vi "Compare to masks.vi"(7 "Number of Particles1":i32=10, 8 "error in (no error)":errorcluster, 9 "Number of Particles":i32=1, 10 "Mask array":T1[](array[typedef]), 11 "Image Src":T1=refnum) -> (0 "Final error out":errorcluster={"status"=TRUE, "code"=-1074395995, "source"=""}, 3 "Marked Regions":bool[](array[boolean]))   [LabVIEW 2009]
doc: "From the marked regions, this VI outputs a one dimensional array of integers. Each element is a sector with a sick distance value in it. The 0th element represents the sector at 180 degrees, whlie the 29th element represents the sector at 0 degrees"
uses:
  <vilib>/vision/Image Controls.llb/IMAQ Image.ctl
  <vilib>/vision/NI_Vision_Development_Module.lvlib
panel:
  out "x < 0?":bool
  out "Erosion iteration":i32=3
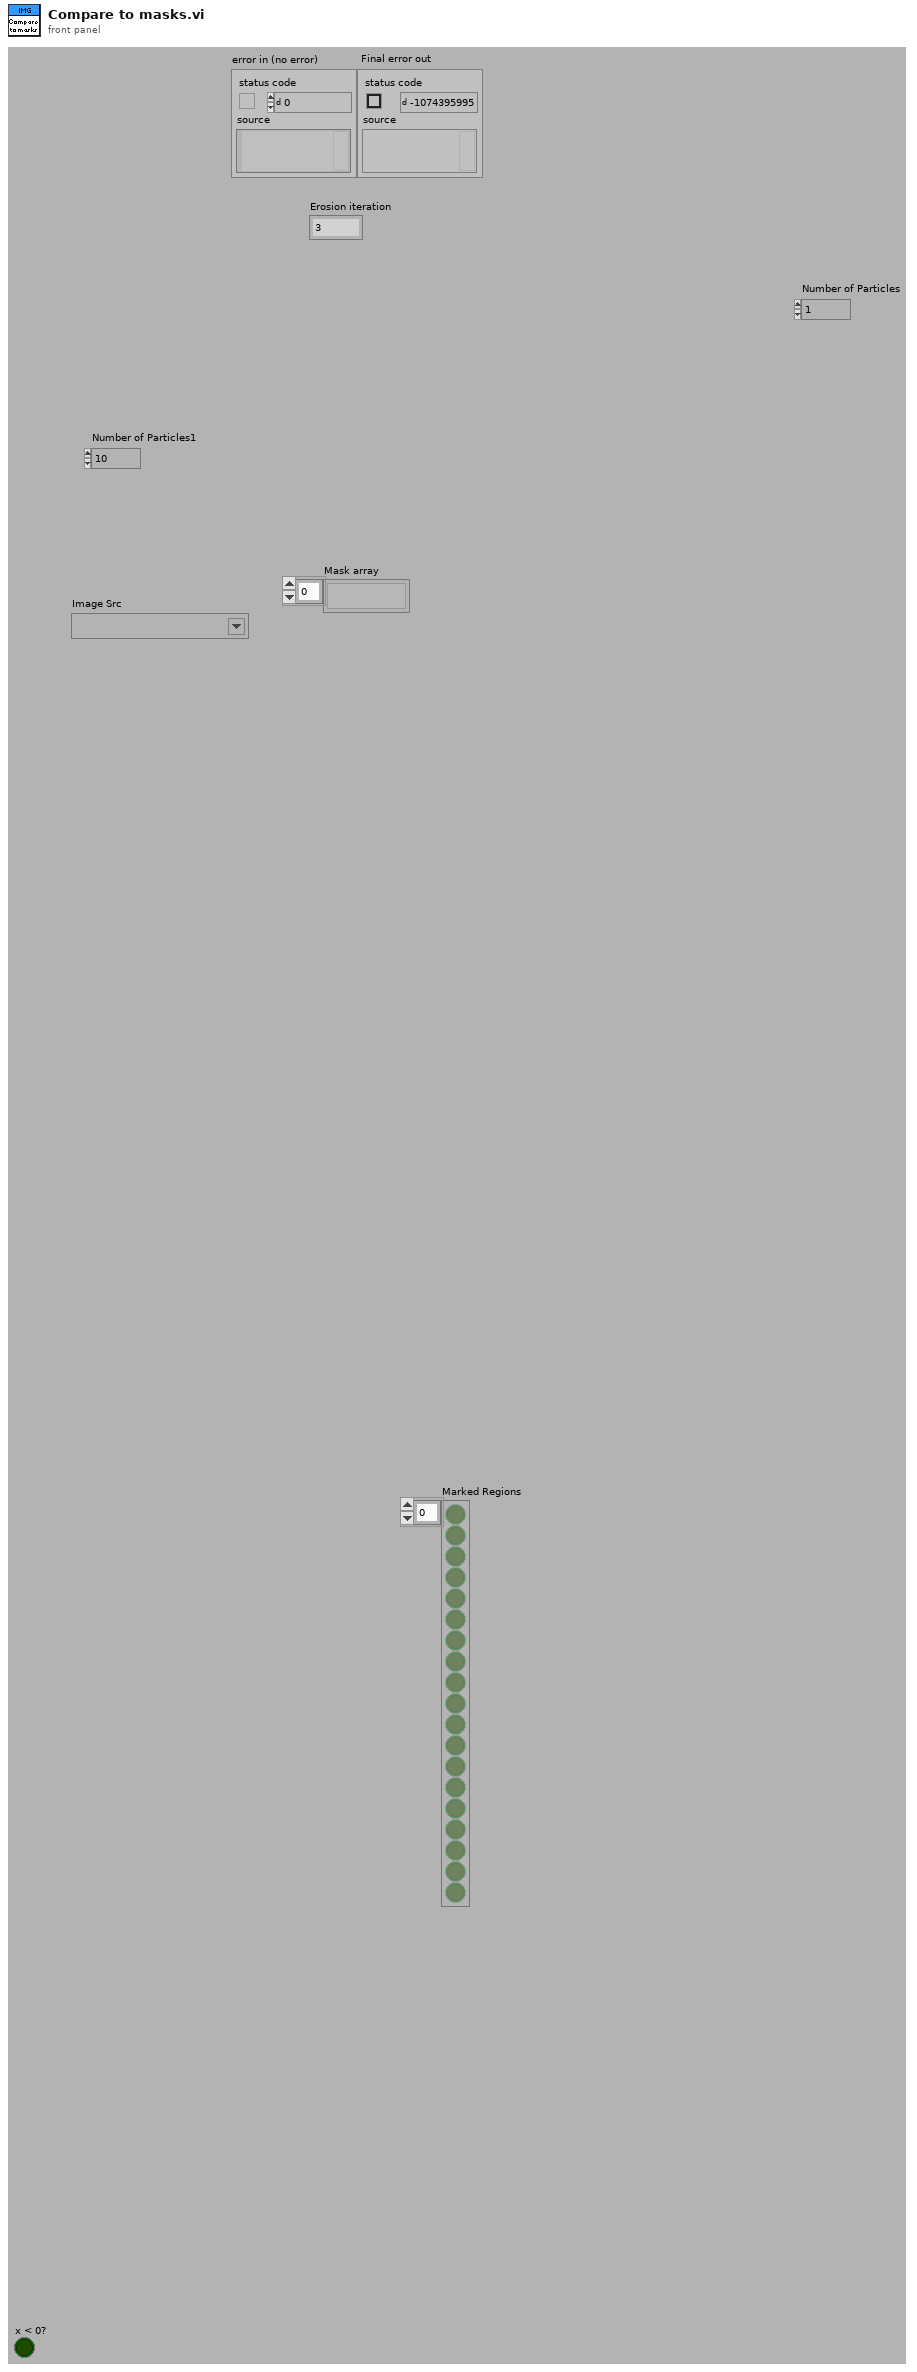
[diagram p1: front panel]
types:
  T1 = typedef "IMAQ Image.ctl" = refnum<image>
  T2 = enum32{"AutoM", "Close", "Dilate", "Erode", "Gradient", "Gradient out", "Gradient in", "Hit miss", "Open", "PClose", "POpen", "Thick", "Thin"}
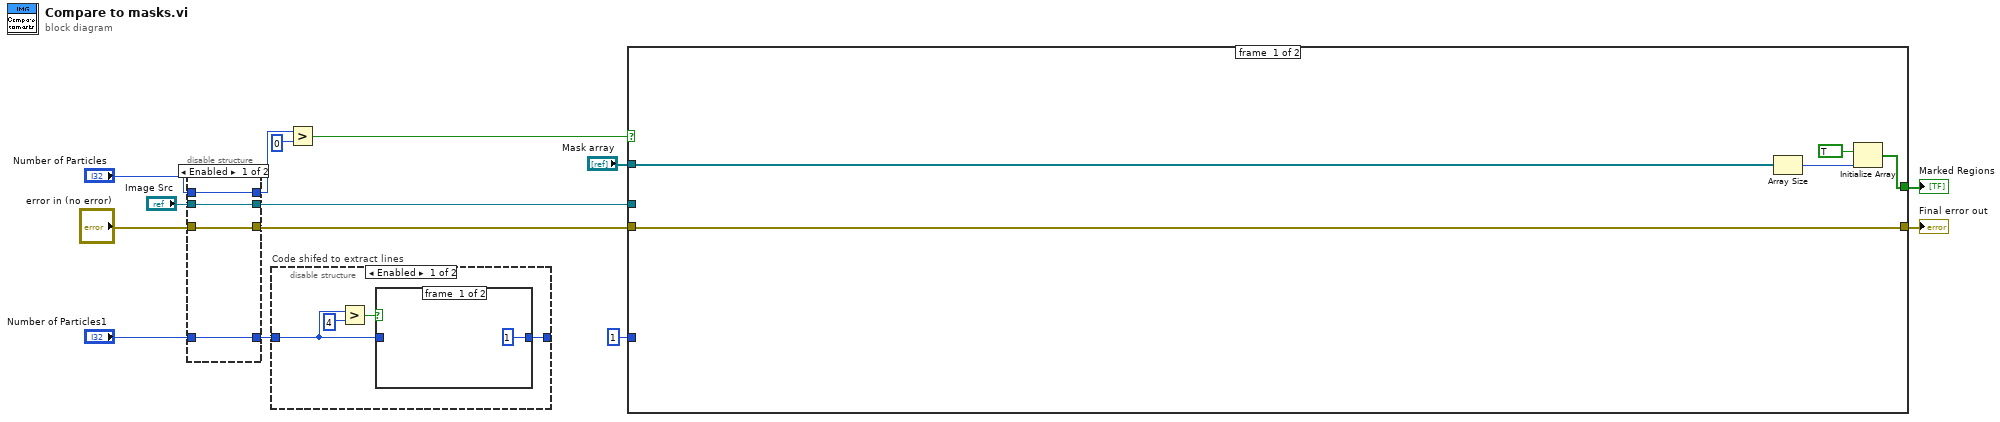
[diagram p0: block diagram]
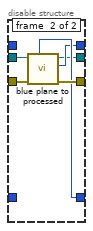
[diagram p2: hidden frame]
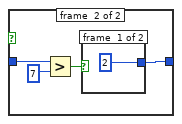
[diagram p3: hidden frame]
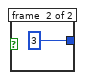
[diagram p4: hidden frame]
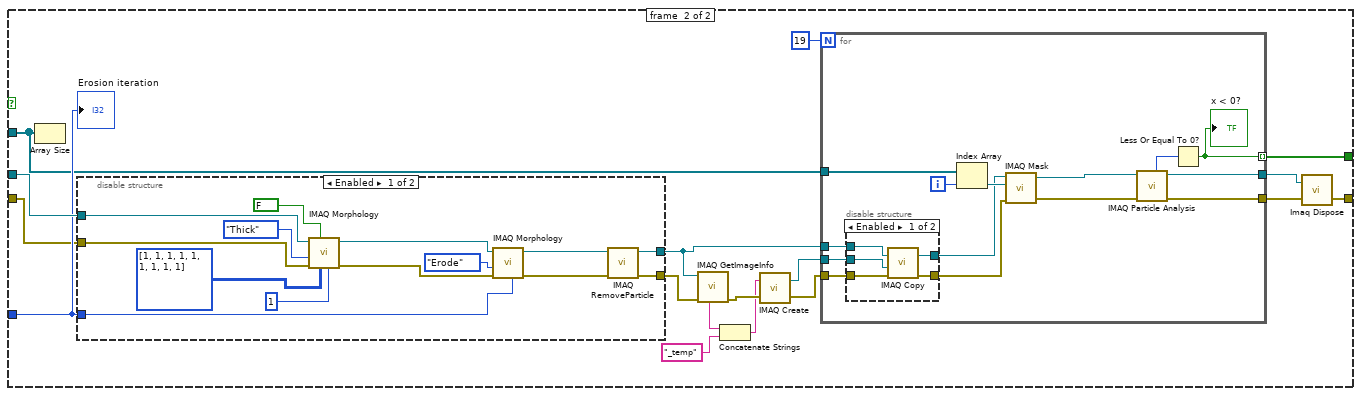
[diagram p6: hidden frame]
diagram:
  n1 = disable-structure shown="Enabled" {
    disable-tunnel: "error in (no error)" -> [w18 w24]
    disable-tunnel: [w18 w23] -> w9
    disable-tunnel: "Image Src" -> [w17 w22]
    disable-tunnel: [w17 w19] -> w2
    disable-tunnel: "Number of Particles" -> [w16 _]
    disable-tunnel: [w16 w20] -> w7
    disable-tunnel: [w15 w21] -> w6
    disable-tunnel: "Number of Particles1" -> [w15 _]
    frame #0 {
    }
    frame #1 {
      n2 = call "blue plane to processed.vi"("error in (no error)"=w24, "Image Src"=w22) -> ("error out"=w23:errorcluster, "Number of Particles"=w20:i32, "Image Dst Out"=w19:T1, "Number of Particles1"=w21:i32)  [unwired: 6 out]
    }
  }
  n3 = disable-structure "Code shifed to extract lines" shown="Enabled" {
    disable-tunnel: [w26 w36] -> _
    disable-tunnel: w6 -> [w25 w36]
    frame #0 {
      n4 = Greater?(x=w25, y=4) -> (0:w27:bool)
      n5 = case shown="True" w27 {
        tunnel: [1 ("Number of iterations (1)") w31] -> w26
        tunnel: w25 -> [_ w33]
        frame #0 {
        }
        frame #1 {
          n6 = Greater?(x=w33, y=7) -> (0:w30:bool)
          n7 = case shown="True" w30 {
            tunnel: [2 ("Number of iterations (1)") 3 ("Number of iterations (1)")] -> w31
            frame #0 {
            }
            frame #1 {
            }
          }
        }
      }
    }
    frame #1 {
    }
  }
  n8 = Greater?(x=w7, y=0) -> (0:w14:bool)
  n9 = case shown="True" w14 {
    tunnel: w2 -> [_ w58]
    tunnel: w9 -> [w41 w55]
    tunnel: 1 ("Number of iterations (1)") -> [_ w57]
    tunnel: [w41 w53] -> w12
    tunnel: "Mask array" -> [w40 w56]
    tunnel: [w37 w52] -> w4
    frame #0 {
      n10 = Array Size(array=w40) -> (size(s)=w39:i32)
      n11 = Initialize Array(TRUE, w39) -> (w37:bool[])
    }
    frame #1 {
      n12 = Array Size(array=w56) -> ()  [unwired: 1 out]
      n13 = disable-structure shown="Enabled" {
        disable-tunnel: w58 -> [w69 w74]
        disable-tunnel: [w63 w74] -> w49
        disable-tunnel: w57 -> [w62 _]
        disable-tunnel: w55 -> [w60 w73]
        disable-tunnel: [w59 w73] -> w48
        frame #0 {
          n14 = call "IMAQ Morphology"("Number of iterations (1)"=1, "Structuring Element"=i32[][] [[1, 1, 1], [1, 1, 1], [1, 1, 1]], "Square/Hexa (Square)"=FALSE, "error in (no error)"=w60, "Operation"=T2."Thick", "Image Src"=w69) -> ("error out"=w67:errorcluster, "Image Dst Out"=w66:T1)  [unwired: 1 in, 3 out]
          n15 = call "IMAQ Morphology"("Number of iterations (1)"=w62, "error in (no error)"=w67, "Operation"=T2."Erode", "Image Src"=w66) -> ("error out"=w65:errorcluster, "Image Dst Out"=w64:T1)  [unwired: 3 in, 3 out]
          n16 = call "IMAQ RemoveParticle"("error in (no error)"=w65, "Image Src"=w64) -> ("error out"=w59:errorcluster, "Image Dst Out"=w63:T1)  [unwired: 5 in, 3 out]
        }
        frame #1 {
        }
      }
      n17 = call "IMAQ GetImageInfo"("error in (no error)"=w48, "Image"=w49) -> ("error out"=w47:errorcluster, "Image Name"=w46:string)  [unwired: 2 in, 6 out]
      n18 = Concatenate Strings(w46, "_temp" ("string")) -> (w44:string)
      n19 = call "IMAQ Create"("Image Name"=w44, "error in (no error)"=w47) -> ("New Image"=w43:T1, "error out"=w42:errorcluster)  [unwired: 3 in]
      n20 = for {
        N: 19 -> [_]
        tunnel: w49 -> [w86]
        tunnel: w56 -> [w85]
        tunnel: w42 -> [w84]
        tunnel: w43 -> [w83]
        tunnel: [w82] -> w54
        tunnel: [w78] -> w50
        tunnel: [w81] -> w52 mode=indexing
        i -> [w80]
        n21 = disable-structure shown="Enabled" {
          disable-tunnel: [w93 w94] -> w87
          disable-tunnel: w86 -> [w92 w95]
          disable-tunnel: w84 -> [w91 w94]
          disable-tunnel: w83 -> [w90 _]
          disable-tunnel: [w89 w95] -> w77
          frame #0 {
            n22 = call "IMAQ Copy"("error in (no error)"=w91, "Image Dst"=w90, "Image Src"=w92) -> ("error out"=w93:errorcluster, "Image Dst Out"=w89:T1)  [unwired: 3 out]
          }
          frame #1 {
          }
        }
        n23 = Index Array(array=w85, index=w80) -> (element=w79:T1)
        n24 = call "IMAQ Mask"("error in (no error)"=w87, "Image Mask"=w79, "Image Src"=w77) -> ("error out"=w75:errorcluster, "Image Dst Out"=w76:T1)  [unwired: 1 in, 1 out]
        n25 = call "IMAQ Particle Analysis"("error in (no error)"=w75, "Image"=w76) -> ("error out"=w82:errorcluster, "Image Out (duplicate)"=w78:T1, "Number of Particles"=w88:i32)  [unwired: 3 in, 4 out]
        n26 = Less Or Equal To 0?(x=w88) -> (x <= 0?=w81:bool)
        "x < 0?" <- w81
      }
      n27 = call "Imaq Dispose"("Image"=w50, "error in (no error)"=w54) -> ("error out"=w53:errorcluster)  [unwired: 4 in]
      "Erosion iteration" <- w57
    }
  }
  "Final error out" <- w12
  "Marked Regions" <- w4
